vi "Results to Waveforms (ddt).vi"(1 "data type":dynamicdata(graph), 7 "result references":T1[](array[typedef]), 11 "error in (no error)":errorcluster) -> (6 "signals out":dynamicdata(graph), 8 "result references out":T1[](array[typedef]), 15 "error out":errorcluster)   [LabVIEW 2020, in "NI_DataFinder.lvlib"]
doc: "Extracts the signals from the results of a DataFinder search."
uses:
  <vilib>/DataFinder/NI_DataFinder.lvlib
  <vilib>/userdefined/DFSearchResult.ctl
  <vilib>/userdefined/NI_DataFinder Controls.lvlib
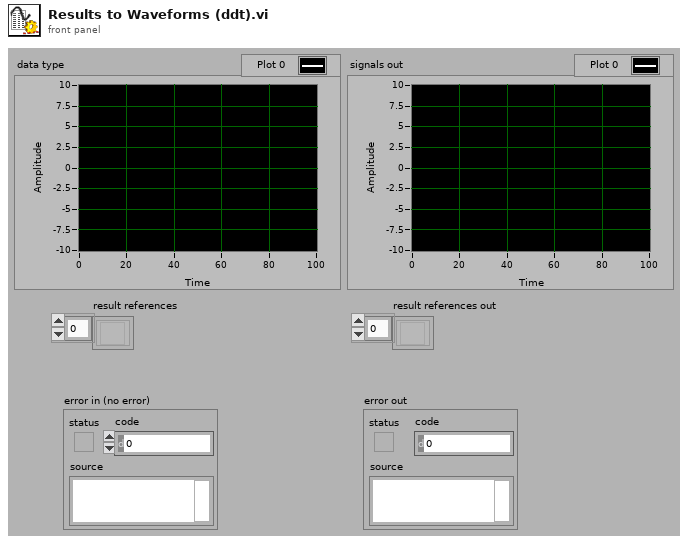
[diagram p1: front panel]
types:
  T1 = typedef "NI_DataFinder Controls.lvlib/DFSearchResult.ctl" = refnum<k20>
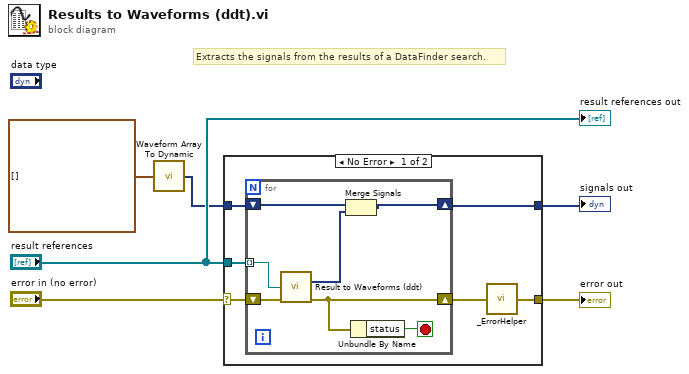
[diagram p0: block diagram]
diagram:
  # "Extracts the signals from the results of a DataFinder search."
  n1 = call <vilib>:"Waveform Array To Dynamic.vi"("Input"=waveform(dbl)[] []) -> ("Output"=w2:dynamicdata)  [unwired: 4 out]
  n2 = case shown="No Error" "error in (no error)" {
    selector: "error in (no error)" -> [w11 w20]
    tunnel: "result references" -> [w12 _]
    tunnel: w2 -> [w9 w21]
    tunnel: [w10 w21] -> w3
    tunnel: [w7 w20] -> w4
    frame No Error {
      n3 = for {
        tunnel: w12 -> [w19] mode=indexing
        shift-right: [w14] -> w8
        shift-left: w11 -> [w18]
        shift-right: [w16] -> w10
        shift-left: w9 -> [w17]
        stop <- w15 stop-if-true
        n4 = call <vilib>:"Result to Waveforms (ddt).vi"("result reference"=w19, "error in"=w18) -> ("signals out"=w13:dynamicdata, "error out"=w14:errorcluster)  [unwired: 12 out]
        n5 = Merge Signals(w17, w13) -> (w16:dynamicdata)
        n6 = Unbundle By Name(w14) -> ("status"=w15:bool)
      }
      n7 = call <vilib>:"_ErrorHelper.vi"("error IO"=w8) -> ("error out"=w7:errorcluster)
    }
    frame Error {
    }
  }
  "error out" <- w4
  "signals out" <- w3
  "result references out" <- "result references"
